vi "cw_1_3.vi"() -> ()   [LabVIEW 2022 SP3]
panel:
  out "Seconds":i32
  out "Minutes":i32
  out "Hours":i32
  out "Days":i32
  out "Weeks":i32
  in  "Seconds":i32
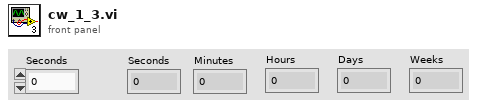
[diagram p1: front panel]
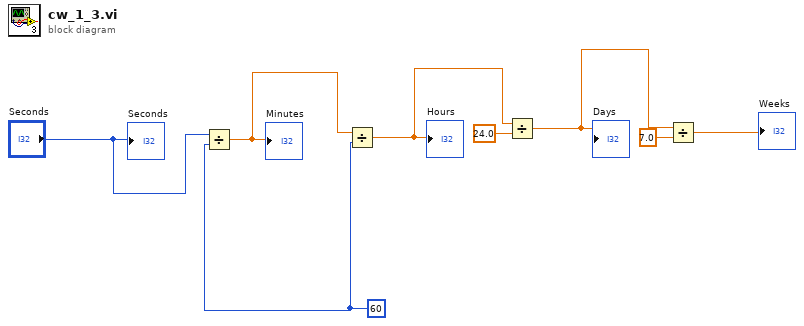
[diagram p0: block diagram]
diagram:
  w3 = 60
  n1 = Divide(x="Seconds", y=w3) -> (x/y=w7:dbl)
  "Minutes" <- w7
  n2 = Divide(x=w7, y=w3) -> (x/y=w6:dbl)
  "Hours" <- w6
  n3 = Divide(x=w6, y=24.0) -> (x/y=w5:dbl)
  "Days" <- w5
  n4 = Divide(x=w5, y=7.0) -> (x/y=→"Weeks":dbl)
  "Seconds" <- "Seconds"
